vi "SetClassQueue.vi"(8 "ErrorIn(No Error)":errorcluster caption="entrée d'erreur (pas d'erreur)", 10 "Menu déroulant":T1 items=["UpdateClassData", "UpdateMainClass"], 11 "Symphony.lvclass":refnum<class "SymphonyCCD.lvclass">) -> (0 "sortie d'erreur":errorcluster, 3 "Symphony.lvclass Out":refnum<class "SymphonyCCD.lvclass">)   [LabVIEW 2019, in "SymphonyCCD.lvclass"]
uses:
  SymphonyCCD.lvclass
  BaseDevice/ClassQueueMess.ctl
  BaseDevice/BaseDevice.lvclass
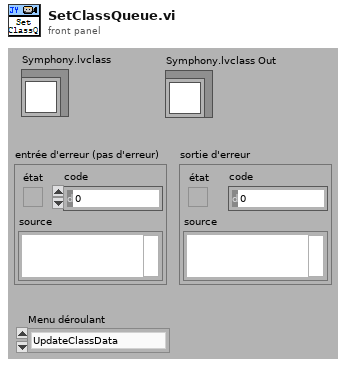
[diagram p1: front panel]
types:
  T1 = typedef "ClassQueueMess.ctl" = u16
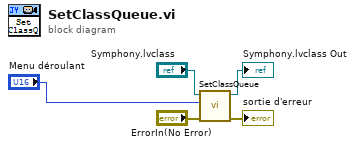
[diagram p0: block diagram]
diagram:
  n1 = call-parent "SetClassQueue.vi"("ErrorIn(No Error)"="ErrorIn(No Error)", "Menu déroulant"="Menu déroulant", "BaseDevice.lvclass"="Symphony.lvclass") -> ("sortie d'erreur"=→"sortie d'erreur":errorcluster, "BaseDevice.lvclass Out"=→"Symphony.lvclass Out":refnum<class "SymphonyCCD.lvclass">)  [unwired: 7 in]
